vi "SplitDouble.vi"(11 "number":dbl) -> (0 "Low":i16, 3 "High":i16)   [LabVIEW 2024]
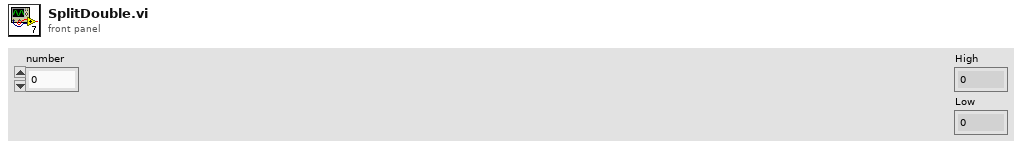
[diagram p1: front panel]
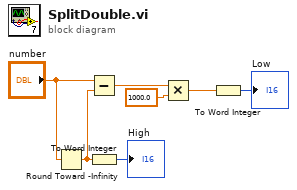
[diagram p0: block diagram]
diagram:
  n1 = Round Toward -Infinity(1:"number") -> (0:w4:dbl)
  n2 = Subtract(x="number", y=w4) -> (x-y=w3:dbl)
  n3 = To Word Integer(number=w4) -> (16bit integer=→"High":i16)
  n4 = Multiply(x=w3, y=1000.0) -> (x*y=w1:dbl)
  n5 = To Word Integer(number=w1) -> (16bit integer=→"Low":i16)
